vi "S2C_PCIe1762H_Proc_DigitalRead.vi"(8 "Error In":errorcluster, 11 "FootSwitch":string) -> (0 "Error Out":errorcluster, 3 "Result":string)   [LabVIEW 2024]
uses:
  TypeDefs/S2C_PCIe1762H_Type_FootSwitch.ctl
  S2C_PCIe1762H_Proc_Globals.vi
  <userlib>/DAQNavi Polymorphic VI/create/DAQNavi Create Channel(DO-Digital Output).vi
  <userlib>/DAQNavi Polymorphic VI/read/DAQNavi Read (Digital U8 1Chan 1Samp).vi
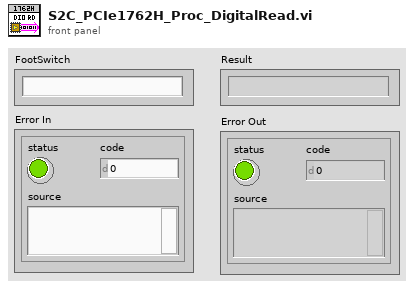
[diagram p1: front panel]
types:
  T1 = typedef "S2C_PCIe1762H_Type_FootSwitch.ctl" = u16
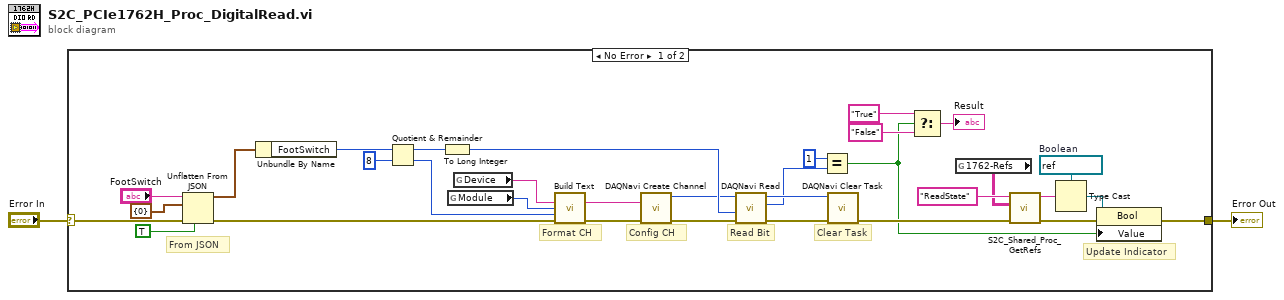
[diagram p0: block diagram]
diagram:
  n1 = case shown="No Error" "Error In" {
    selector: "Error In" -> [w18 w36]
    tunnel: [w6 w36] -> w1
    frame No Error {
      w8 = refnum<vi> refnum  # Boolean
      # "Update Indicator"
      # "Clear Task"
      # "Read Bit"
      # "Format CH"
      # "Config CH"
      # "From JSON"
      n2 = Unflatten From JSON(JSON string="FootSwitch", type and defaults=cluster{"FootSwitch":T1} {"FootSwitch"=0}, default null elements? (F)=TRUE, error in (no error)=w18) -> (value=w32:cluster{"FootSwitch":T1}, error out=w31:errorcluster)  [unwired: 3 in]
      n3 = Unbundle By Name(w32) -> ("FootSwitch"=w30:T1)
      n4 = Quotient & Remainder(x=w30, y=u16 8) -> (x-y*floor(x/y)=w25:T1, floor(x/y)=w26:T1)
      n5 = To Long Integer(number=w25) -> (32bit integer=w24:i32)
      n6 = global read "S2C_PCIe1762H_Proc_Globals.vi" "Module"() -> (w17:i32)
      n7 = global read "S2C_PCIe1762H_Proc_Globals.vi" "Device"() -> (w16:string)
      n8 = call "Build Text"("Device"=w16, "Module"=w17, "Port"=w26, "error in (no error)"=w31) -> ("Result"=w27:string, "error out"=w28:errorcluster)  [unwired: 10 in]
      n9 = call-poly <userlib>:"DAQNavi Create Channel.vi"("physical channels"=w27, "error in (no error)"=w28) -> ("task out"=w14:i32, "error out"=w15:errorcluster)  [unwired: 3 in, 9 out]
      n10 = call-poly <userlib>:"DAQNavi Read.vi"("error in (no error)"=w15, "portBit"=w24, "task in"=w14) -> ("error out"=w23:errorcluster, "data"=w13:u8, "task out"=w22:i32)  [unwired: 1 in, 5 out]
      n11 = Equal?(x=u8 1, y=w13) -> (x = y?=w4:bool)
      n12 = call <userlib>:"DAQNavi Clear Task.vi"("error in (no error)"=w23, "task in"=w22) -> ("error out"=w5:errorcluster)  [unwired: 1 out]
      n13 = Select(t="True", s=w4, f="False") -> (s? t:f=→"Result":string)
      n14 = global read "S2C_PCIe1762H_Proc_Globals.vi" "1762-Refs"() -> (w3:string[][])
      n15 = call "S2C_Shared_Proc_GetRefs.vi"("Error In"=w5, "Refs"=w3, "Label"="ReadState") -> ("Error Out"=w10:errorcluster, "Reference"=w9:string)  [unwired: 7 in]
      n16 = Type Cast(type=w8, x=w9) -> (*(type *) &x=w11:refnum<vi>)
      n17 = property class="Bool"(reference=w11, error in=w10, "Value"=w4) -> (error out=w6:errorcluster)  [unwired: 1 out]
    }
    frame Error {
    }
  }
  "Error Out" <- w1
